vi "Calibration (SubVI).vi"(7 "VISA UUT":refnum<visa-resource-name>="COM6", 8 "error constant":errorcluster, 9 "UUT":refnum<vi>, 10 "CAN Cluster in":refnum<vi>, 11 "Visa Tester":refnum<vi>) -> (0 "error constant 2":errorcluster, 2 "AO[1]Meas":dbl)   [LabVIEW 2017]
panel:
  out "Ope":T1(array[ring])=[enum."0C", enum."10C", enum."20C", enum."25C", enum."30C", enum."40C", enum."50C", enum."60C", enum."70C", enum."80C", enum."90C", enum."100C", enum."110C", enum."120C"]
  in  "OK Button":bool
  in  "Boolean 14":bool
  in  "Boolean 13":bool
  in  "Boolean 12":bool
  in  "Boolean 11":bool
  in  "Boolean 10":bool
  in  "Boolean 9":bool
  in  "Boolean 8":bool
  in  "Boolean 7":bool
  in  "Boolean 6":bool
  in  "Boolean 5":bool
  in  "Boolean 4":bool
  in  "Boolean 3":bool
  in  "Boolean 2":bool
  in  "Boolean":bool
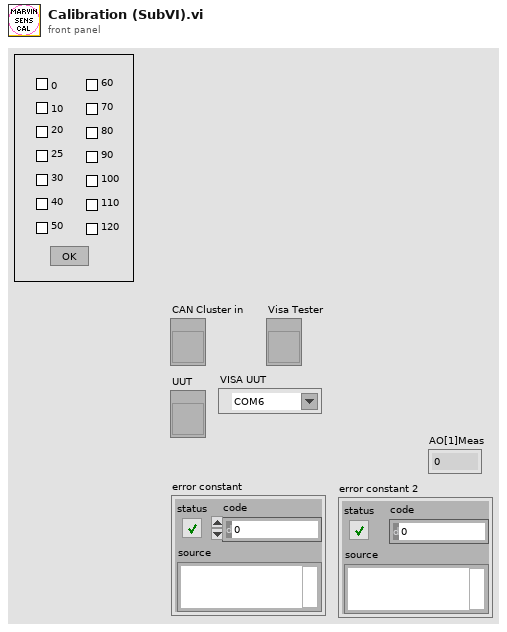
[diagram p1: front panel]
types:
  T1 = enum16{"K15", "K16", "K17", "Venable", "Firmeware", "Fan", "Power", "120C", "110C", "100C", "90C", "80C", "70C", "60C", "50C", "40C", "30C", "25C", "20C", "10C", "0C"}[]
  T2 = enum16{"Stop", "AO[1]=Meas.", "TA[5]", "AO[1]=0", "Start"}
  T3 = enum32{"Invalid", "Standard", "Closed", "Hidden", "Minimized", "Maximized"}
  T4 = enum16{"K15", "K16", "K17", "Venable", "Firmeware", "Fan", "Power", "120C", "110C", "100C", "90C", "80C", "70C", "60C", "50C", "40C", "30C", "25C", "20C", "10C", "0C"}
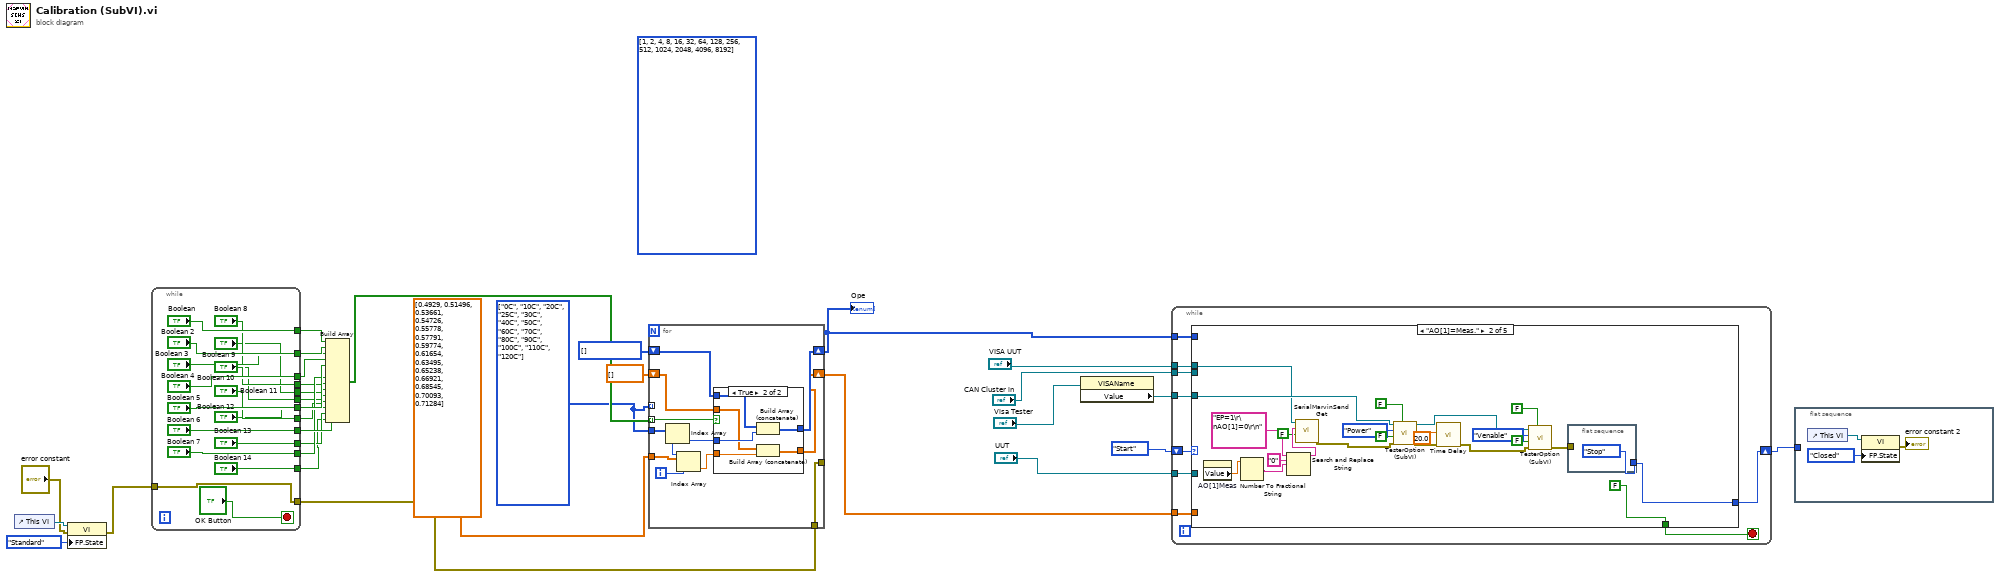
[diagram p0: block diagram]
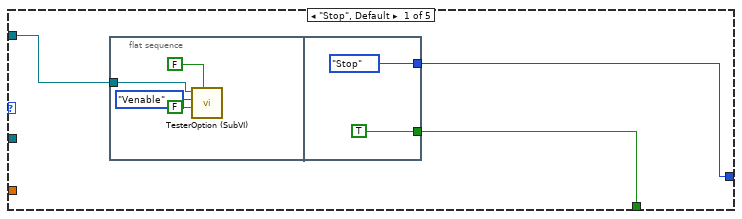
[diagram p2: hidden frame]
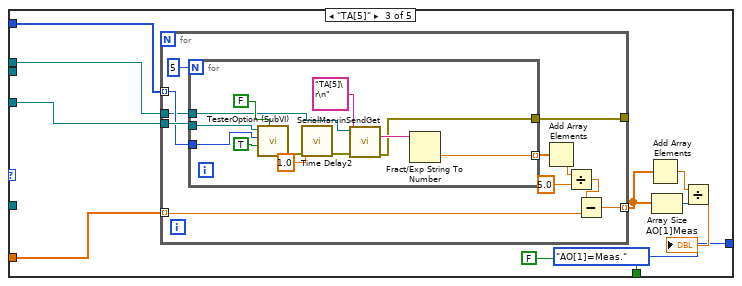
[diagram p3: hidden frame]
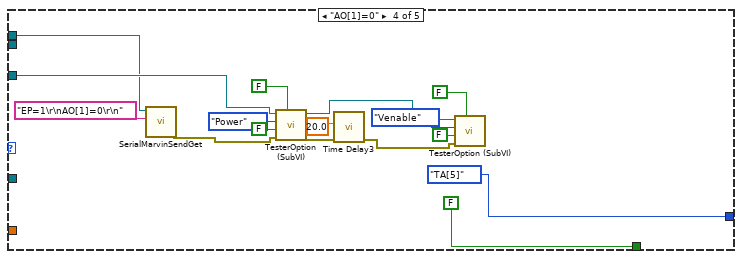
[diagram p4: hidden frame]
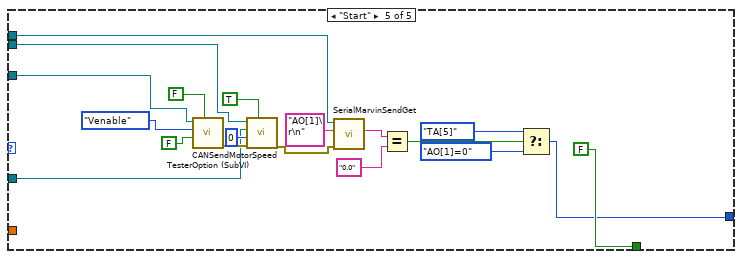
[diagram p5: hidden frame]
diagram:
  w4 = T1 [] items=["K15", "K16", "K17", "Venable", "Firmeware", "Fan", "Power", "120C", "110C", "100C", "90C", "80C", "70C", "60C", "50C", "40C", "30C", "25C", "20C", "10C", "0C"]
  w6 = T1 [enum."0C", enum."10C", enum."20C", enum."25C", enum."30C", enum."40C", enum."50C", enum."60C", enum."70C", enum."80C", enum."90C", enum."100C", enum."110C", enum."120C"] items=["K15", "K16", "K17", "Venable", "Firmeware", "Fan", "Power", "120C", "110C", "100C", "90C", "80C", "70C", "60C", "50C", "40C", "30C", "25C", "20C", "10C", "0C"]
  (unwired) u32[] [1, 2, 4, 8, 16, 32, 64, 128, 256, 512, 1024, 2048, 4096, 8192] ("appended array")
  n1 = control-ref of="This VI"() -> (w15:refnum<vi>)
  n2 = property class="VI"(reference=w15, error in="error constant", "FP.State"=T3."Standard" ("Front Panel Window:State")) -> (error out=w12:errorcluster)  [unwired: 1 out]
  n3 = while {
    tunnel: ["Boolean"] -> w31
    tunnel: ["Boolean 2"] -> w30
    tunnel: ["Boolean 3"] -> w29
    tunnel: ["Boolean 4"] -> w28
    tunnel: ["Boolean 5"] -> w27
    tunnel: ["Boolean 6"] -> w26
    tunnel: ["Boolean 7"] -> w25
    tunnel: ["Boolean 8"] -> w24
    tunnel: ["Boolean 9"] -> w23
    tunnel: ["Boolean 10"] -> w22
    tunnel: ["Boolean 11"] -> w21
    tunnel: ["Boolean 12"] -> w20
    tunnel: ["Boolean 13"] -> w19
    tunnel: ["Boolean 14"] -> w18
    tunnel: [w34] -> w14
    tunnel: w12 -> [w34]
    stop <- "OK Button" stop-if-true
  }
  n4 = Build Array(w31, w30, w29, w28, w27, w26, w25, w24, w23, w22, w21, w20, w19, w18) -> (w17:bool[])
  n5 = for {
    tunnel: w6 -> [_] mode=indexing
    tunnel: w6 -> [w60]
    tunnel: dbl[] [0.4929, 0.51496, 0.53661, 0.54726, 0.55778, 0.57791, 0.59774, 0.61654, 0.63495, 0.65238, 0.66921, 0.68545, 0.70093, 0.71284] -> [w59]
    shift-right: [w53] -> w5
    shift-left: w4 -> [w55]
    shift-right: [w52] -> w7
    shift-left: dbl[] [] -> [w54]
    tunnel: w17 -> [w51] mode=indexing
    tunnel: [w50] -> _
    tunnel: w14 -> [w50]
    i -> [w58]
    n6 = Index Array(array=w60, index=w58) -> (element=w56:T4)
    n7 = Index Array(array=w59, index=w58) -> (element=w57:dbl)
    n8 = case shown="True" w51 {
      tunnel: w57 -> [_ w64]
      tunnel: w56 -> [_ w67]
      tunnel: w55 -> [w62 w68]
      tunnel: w54 -> [w61 w65]
      tunnel: [w62 w66] -> w53
      tunnel: [w61 w63] -> w52
      frame False {
      }
      frame True {
        n9 = Build Array (concatenate)(w68, w67) -> (w66:T1)
        n10 = Build Array (concatenate)(w65, w64) -> (w63:dbl[])
      }
    }
  }
  "Ope" <- w5
  n11 = property on="Property Node" class="VISAName"(reference="Visa Tester") -> ("Value"=w2:refnum<visa-resource-name>)  [unwired: 1 in, 2 out]
  n12 = while {
    shift-right: [w75] -> w1
    shift-left: T2."Start" -> [w77]
    tunnel: w2 -> [w76]
    tunnel: "CAN Cluster in" -> [w69]
    tunnel: "UUT" -> [w73]
    tunnel: "VISA UUT" -> [w72]
    tunnel: w7 -> [w71]
    tunnel: w5 -> [w70]
    stop <- w74 stop-if-true
    n13 = case shown="\"AO[1]=Meas.\"" w77 {
      tunnel: w76 -> [w80 w104 w119 w153 w163]
      tunnel: [w78 w91 T2."AO[1]=Meas." ("f") T2."TA[5]" ("f") w160] -> w75
      tunnel: [w79 FALSE FALSE FALSE FALSE] -> w74
      tunnel: w73 -> [_ _ _ _ w162]
      tunnel: w72 -> [_ w87 w110 w143 w161]
      tunnel: w71 -> [_ _ w115 _ _]
      tunnel: w70 -> [_ _ w112 _ _]
      tunnel: w69 -> [_ _ _ _ w159]
      frame "Stop", Default {
        n14 = flat-sequence {
          tunnel: w80 -> [w81]
          tunnel: [TRUE] -> w79
          tunnel: [T2."Stop"] -> w78
          frame #0 {
            n15 = call "TesterOption (SubVI).vi"("2 Options"=FALSE, "On/Off"=FALSE, "Tester Option"=T4."Venable", "VISA Refnum in"=w81) -> ()  [unwired: 6 in, 2 out]
          }
          frame #1 {
          }
        }
      }
      frame "AO[1]=Meas." {
        n16 = property on="AO[1]Meas" class="DigNum (strict)"() -> ("Value"=w90:dbl)  [unwired: 2 in, 2 out]
        n17 = Number To Fractional String(number=w90) -> (F-format string=w93:string)  [unwired: 3 in]
        n18 = Search and Replace String(input string="EP=1\r\nAO[1]=0\r\n" ("write buffer"), search string="0", replace string=w93) -> (result string=w92:string)  [unwired: 5 in, 3 out]
        n19 = call "SerialMarvinSendGet.vi"("Clear Log"=FALSE, "write buffer"=w92, "VISA resource name"=w87) -> ("error out"=w103:errorcluster)  [unwired: 7 in, 1 out]
        n20 = call "TesterOption (SubVI).vi"("2 Options"=FALSE, "error in (no error)"=w103, "On/Off"=FALSE, "Tester Option"=T4."Power", "VISA Refnum in"=w104) -> ("error out"=w102:errorcluster, "VISA Refnum out"=w96:refnum<visa-resource-name>)  [unwired: 5 in]
        n21 = call "Time Delay"("error in (no error)"=w102, "Delay Time (s)"=20.0 ("Time to wait")) -> ("error out"=w97:errorcluster)  [unwired: 9 in]
        n22 = call "TesterOption (SubVI).vi"("2 Options"=FALSE, "error in (no error)"=w97, "On/Off"=FALSE, "Tester Option"=T4."Venable", "VISA Refnum in"=w96) -> ("error out"=w89:errorcluster)  [unwired: 5 in, 1 out]
        n23 = flat-sequence {
          tunnel: [T2."Stop"] -> w91
          tunnel: w89 -> [_]
          frame #0 {
          }
        }
      }
      frame "TA[5]" {
        n24 = for {
          tunnel: w119 -> [w129]
          tunnel: w115 -> [w124] mode=indexing
          tunnel: [w123] -> w114 mode=indexing
          tunnel: [w122] -> _
          tunnel: w112 -> [w121] mode=indexing
          tunnel: w110 -> [w120]
          n25 = for {
            N: 5 -> [_]
            tunnel: w129 -> [w137]
            tunnel: [w134] -> w128 mode=indexing
            tunnel: [w133] -> w122
            tunnel: w121 -> [w132]
            tunnel: w120 -> [w131]
            n26 = call "TesterOption (SubVI).vi"("2 Options"=FALSE, "On/Off"=TRUE, "Tester Option"=w132, "VISA Refnum in"=w137) -> ("error out"=w138:errorcluster)  [unwired: 6 in, 1 out]
            n27 = call "Time Delay2"("error in (no error)"=w138, "Delay Time (s)"=1.0 ("Time to wait")) -> ("error out"=w136:errorcluster)  [unwired: 9 in]
            n28 = call "SerialMarvinSendGet.vi"("error in (no error)"=w136, "write buffer"="TA[5]\r\n", "VISA resource name"=w131) -> ("error out"=w133:errorcluster, "read buffer"=w139:string)  [unwired: 7 in]
            n29 = Fract/Exp String To Number(string=w139) -> (number=w134:dbl)  [unwired: 3 in, 1 out]
          }
          n30 = Add Array Elements(numeric array=w128) -> (sum=w127:dbl)
          n31 = Divide(x=w127, y=5.0) -> (x/y=w125:dbl)
          n32 = Subtract(x=w125, y=w124) -> (x-y=w123:dbl)
        }
        n33 = Add Array Elements(numeric array=w114) -> (sum=w117:dbl)
        n34 = Array Size(array=w114) -> (size(s)=w113:i32)
        n35 = Divide(x=w117, y=w113) -> (x/y=→"AO[1]Meas":dbl)
      }
      frame "AO[1]=0" {
        n36 = call "SerialMarvinSendGet.vi"("write buffer"="EP=1\r\nAO[1]=0\r\n", "VISA resource name"=w143) -> ("error out"=w152:errorcluster)  [unwired: 8 in, 1 out]
        n37 = call "TesterOption (SubVI).vi"("2 Options"=FALSE, "error in (no error)"=w152, "On/Off"=FALSE, "Tester Option"=T4."Power", "VISA Refnum in"=w153) -> ("error out"=w151:errorcluster, "VISA Refnum out"=w145:refnum<visa-resource-name>)  [unwired: 5 in]
        n38 = call "Time Delay3"("error in (no error)"=w151, "Delay Time (s)"=20.0 ("Time to wait")) -> ("error out"=w146:errorcluster)  [unwired: 9 in]
        n39 = call "TesterOption (SubVI).vi"("2 Options"=FALSE, "error in (no error)"=w146, "On/Off"=FALSE, "Tester Option"=T4."Venable", "VISA Refnum in"=w145) -> ()  [unwired: 5 in, 2 out]
      }
      frame "Start" {
        n40 = call "TesterOption (SubVI).vi"("2 Options"=FALSE, "On/Off"=FALSE, "Tester Option"=T4."Venable", "VISA Refnum in"=w163) -> ("error out"=w173:errorcluster)  [unwired: 6 in, 1 out]
        n41 = call "CANSendMotorSpeed.vi"("Remote"=TRUE, "error in (no error)"=w173, "Motor Speed RPM"=u16 0, "UUT"=w162, "CAN Cluster in"=w159) -> ("error out"=w170:errorcluster)  [unwired: 6 in]
        n42 = call "SerialMarvinSendGet.vi"("error in (no error)"=w170, "write buffer"="AO[1]\r\n", "VISA resource name"=w161) -> ("read buffer"=w169:string)  [unwired: 7 in, 1 out]
        n43 = Equal?(x=w169, y="0.0") -> (x = y?=w164:bool)
        n44 = Select(t=T2."TA[5]", s=w164, f=T2."AO[1]=0") -> (s? t:f=w160:T2)
      }
    }
  }
  n45 = flat-sequence {
    tunnel: w1 -> [_]
    frame #0 {
      n46 = control-ref of="This VI"() -> (w180:refnum<vi>)
      n47 = property class="VI"(reference=w180, "FP.State"=T3."Closed" ("Front Panel Window:State")) -> (error out=→"error constant 2":errorcluster)  [unwired: 1 in, 1 out]
    }
  }
